vi "InitScreen.vi"(7 "game_screen":refnum<vi>, 8 "error in":errorcluster) -> (0 "error our":errorcluster, 3 "InitCluster_OUT":T1)   [LabVIEW 2019]
uses:
  <vilib>/picture/picture.llb/imagedata.ctl
  ShotInitCluster.ctl
  CharacterCluster.ctl
  InitCluster.ctl
  <vilib>/Utility/miscctls.llb/LVPositionTypeDef.ctl
  <vilib>/Utility/miscctls.llb/LVBoundsTypeDef.ctl
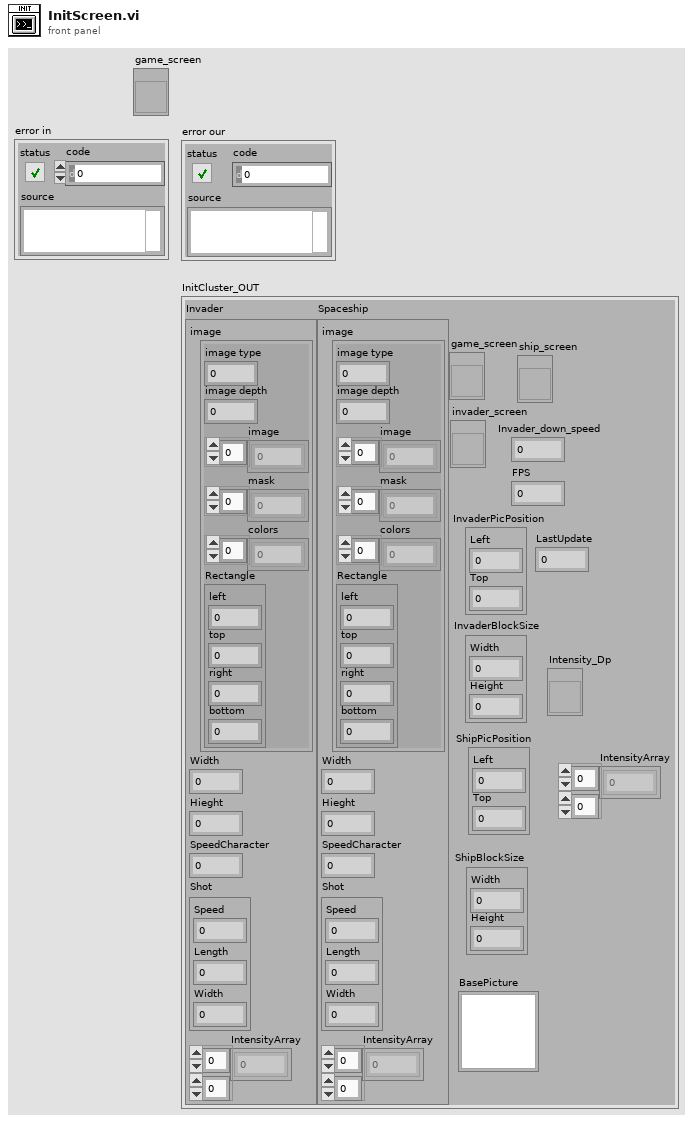
[diagram p1: front panel]
types:
  T1 = typedef "InitCluster.ctl" = cluster{"Invader":T2, "Spaceship":T2, "game_screen":refnum<vi>, "BasePicture":picture, "invader_screen":refnum<vi>, "InvaderPicPosition":T5, "Invader_down_speed":i16, "FPS":u16, "InvaderBlockSize":T6, "ship_screen":refnum<vi>, "ShipBlockSize":T6, "ShipPicPosition":T5, "LastUpdate":u32, "Intensity_Dp":refnum<vi>, "IntensityArray":u8[][]}
  T2 = typedef "CharacterCluster.ctl" = cluster{"image":T3, "Width":u32, "Hieght":u32, "SpeedCharacter":u32, "Shot":T4, "IntensityArray":u8[][]}
  T3 = typedef "imagedata.ctl" = cluster{"image type":i32, "image depth":i32, "image":u8[], "mask":u8[], "colors":u32[], "Rectangle":cluster{"left":i16, "top":i16, "right":i16, "bottom":i16}}
  T4 = typedef "ShotInitCluster.ctl" = cluster{"Speed":u32, "Length":u32, "Width":u32}
  T5 = typedef "LVPositionTypeDef.ctl" = cluster{"Left":i32, "Top":i32}
  T6 = typedef "LVBoundsTypeDef.ctl" = cluster{"Width":u32, "Height":u32}
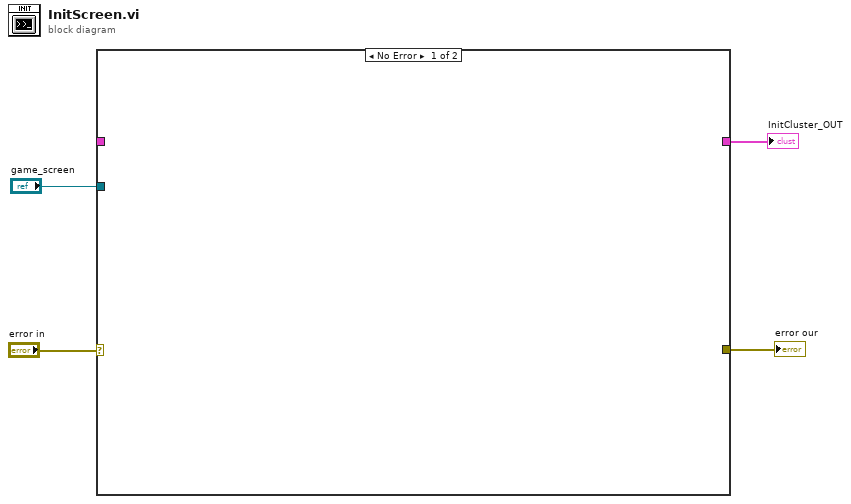
[diagram p0: block diagram]
diagram:
  n1 = case shown="No Error" "error in" {
    selector: "error in" -> [w6 w8]
    tunnel: _ -> [_ w9]
    tunnel: "game_screen" -> [w7 _]
    tunnel: [_ w9] -> w2
    tunnel: [w5 w8] -> w1
    frame No Error {
    }
    frame Error {
    }
  }
  "InitCluster_OUT" <- w2
  "error our" <- w1
